vi "read line from table.vi"(8 "error in":errorcluster, 10 "line number":i32, 11 "operations table":refnum<vi>) -> (0 "error out":errorcluster, 1 "line":T1, 2 "empty tag?":bool, 3 "empty channel?":bool)   [LabVIEW 2013, in "Scan Engine editor node.lvclass"]
uses:
  Scan Engine editor node.lvclass
  table line.ctl
  <vilib>/NI/Tag Bus Module Framework/channel/TBM channel.lvclass
  <vilib>/NI/Tag Bus/tag/tag descriptor.lvclass/tag descriptor.ctl
  <vilib>/NI/Tag Bus/tag/read tag name.vi
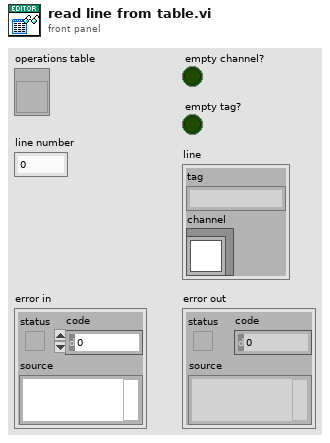
[diagram p1: front panel]
types:
  T1 = typedef "Scan Engine editor node.lvclass/table line.ctl" = cluster{"tag":string, "channel":refnum<class "TBM channel.lvclass">}
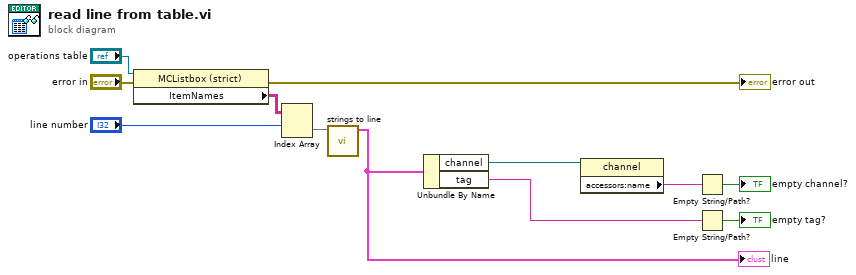
[diagram p0: block diagram]
diagram:
  n1 = property class="MCListbox (strict)"(reference="operations table", error in="error in") -> (error out=→"error out":errorcluster, "ItemNames"=w9:string[][])  [unwired: 1 out]
  n2 = Index Array(array=w9, index (row)="line number") -> (element=w7:string[])  [unwired: 1 in]
  n3 = call "strings to line.vi"("strings"=w7) -> ("line"=w1:T1)  [unwired: 10 in]
  "line" <- w1
  n4 = Unbundle By Name(w1) -> ("channel"=w6:refnum<class "TBM channel.lvclass">, "tag"=w4:string)
  n5 = property class="channel"(reference=w6) -> ("accessors:name"=w5:string)  [unwired: 1 in, 2 out]
  n6 = Empty String/Path?(string/path=w5) -> (empty?=→"empty channel?":bool)
  n7 = Empty String/Path?(string/path=w4) -> (empty?=→"empty tag?":bool)
